vi "Calc XYZ_j.vi"(8 "theta_j":dbl, 9 "j":i32, 11 "Analytical Serial Arm Class in":refnum<class "NI_Robotics_Analytical Serial Arm Class.lvclass">) -> (2 "XYZ_j":dbl[](array[numeric]), 3 "Analytical Serial Arm Class out":refnum<class "NI_Robotics_Analytical Serial Arm Class.lvclass">)   [LabVIEW 2017, in "NI_Robotics_Analytical Serial Arm Class.lvclass"]
uses:
  <vilib>/robotics/Kinematics/Analytical/Generic/NI_Robotics_Analytical Serial Arm Class.lvclass
  c:/Program Files (x86)/National Instruments/LabVIEW 2017/vi.lib/robotics/Kinematics/Robot/NI_Robotics_Serial Robot Arm.lvclass
  <vilib>/robotics/Kinematics/Link/NI_Robotics_Link.lvclass/NI_Robotics_Link.ctl
  <vilib>/robotics/Kinematics/Link/Get Kinematic Parameters.vi
  <vilib>/robotics/Kinematics/Analytical/Generic/Accessors/Read alpha_n0.vi
  <vilib>/robotics/Kinematics/Robot/Get Links.vi
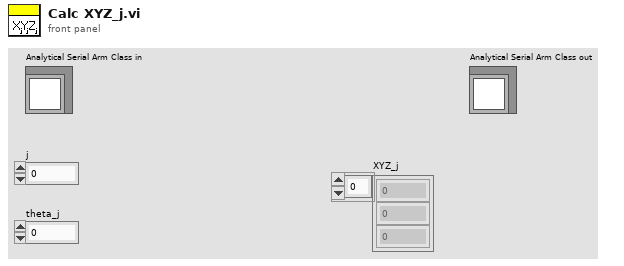
[diagram p1: front panel]
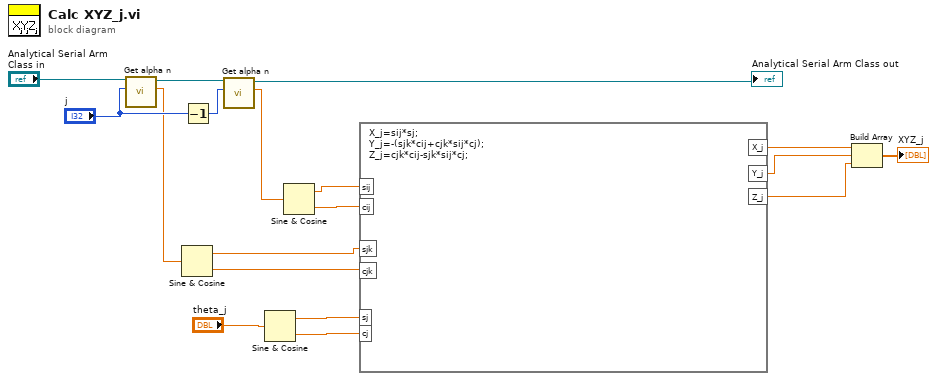
[diagram p0: block diagram]
diagram:
  n1 = call <vilib>:"Get alpha n.vi"("n"="j", "Analytical Serial Arm Class in"="Analytical Serial Arm Class in") -> ("alpha n"=w14:dbl, "Analytical Serial Arm Class out"=w16:refnum<class "NI_Robotics_Analytical Serial Arm Class.lvclass">)  [unwired: 8 in]
  n2 = Sine & Cosine(0:w14) -> (1:w11:dbl, 2:w10:dbl)
  n3 = Decrement(x="j") -> (x-1=w18:i32)
  n4 = call <vilib>:"Get alpha n.vi"("n"=w18, "Analytical Serial Arm Class in"=w16) -> ("alpha n"=w13:dbl, "Analytical Serial Arm Class out"=→"Analytical Serial Arm Class out":refnum<class "NI_Robotics_Analytical Serial Arm Class.lvclass">)  [unwired: 8 in]
  n5 = Sine & Cosine(0:"theta_j") -> (1:w6:dbl, 2:w5:dbl)
  n6 = Sine & Cosine(0:w13) -> (1:w8:dbl, 2:w9:dbl)
  n7 = formula code="X_j=sij*sj;\nY_j=-(sjk*cij+cjk*sij*cj);\nZ_j=cjk*cij-sjk*sij*cj;"("sij"=w8, "cij"=w9, "sjk"=w11, "cjk"=w10, "sj"=w6, "cj"=w5) -> ("X_j"=w4:dbl, "Y_j"=w3:dbl, "Z_j"=w2:dbl)
  n8 = Build Array(w4, w3, w2) -> (→"XYZ_j":dbl[])
